vi "ControlPanelVI.vi"() -> ()   [LabVIEW 2024]
uses:
  <vilib>/Utility/error.llb/Trim Whitespace One-Sided.vi
  <vilib>/Instr/_visa.llb/VISA Configure Serial Port (Instr).vi
  <vilib>/regexp/Match Regular Expression.xnode
panel:
  out "CONTROL PANEL":enum32{" PAGE 1", "SERIAL PORT"}(tab)
  out "DOWN":u32(colorbox)
  out "-----":u32(colorbox)
  out "UP":u32(colorbox)
  out "Waveform Chart":u32(graph)
  out "on/off":u32(colorbox)=56405
  in  "SET ANGLE":i8(slide) min=-90 max=80 step=1 scale=-90.0..80.0
  out "Incline":i8(knob) scale=-90.0..80.0
  out "return count read":u32
  out "READ BUFFER":string
  in  "STOP":bool
  in  "milliseconds to wait":u32=1
  out "return count write":u32
  out "VISA resource name out read":refnum<visa-resource-name>="COM3"
  out "VISA resource name out write":refnum<visa-resource-name>="COM3"
  in  "send msg":bool
  in  "Safe Control":bool=TRUE
  out "input command":i8
  out "PWM (ms)":string
  out "DTC%":u8
  out "error out write":errorcluster
  out "error out read":errorcluster
  in  "VISA resource name":refnum<visa-resource-name>="COM3"
  in  "Enable Termination\nChar (T)":bool=TRUE
  in  "timeout (10sec)":u32=10000
  in  "baud rate (9600)":u32=9600
  in  "byte count":u32=100
  in  "parity (0:none)":enum16{"None", "Odd", "Even", "Mark", "Space"}(ring)
  in  "data bits (8)":u16=8 min=5 max=8 step=1
  in  "termination char\n(0xA = '\\n' = LF)":u8=10 format="%.0x"
  in  "flow control (0:none)":u16(ring)=3 items=["None", "XON/XOFF", "RTS/CTS", "XON/XOFF & RTS/CTS", "DTR/DSR", "XON/XOFF & DTR/DSR"]
  in  "stop bits (10: 1 bit)":u16(ring)=10 items=["1.0"=10, "1.5"=15, "2.0"=20]
  # "per = 20000"
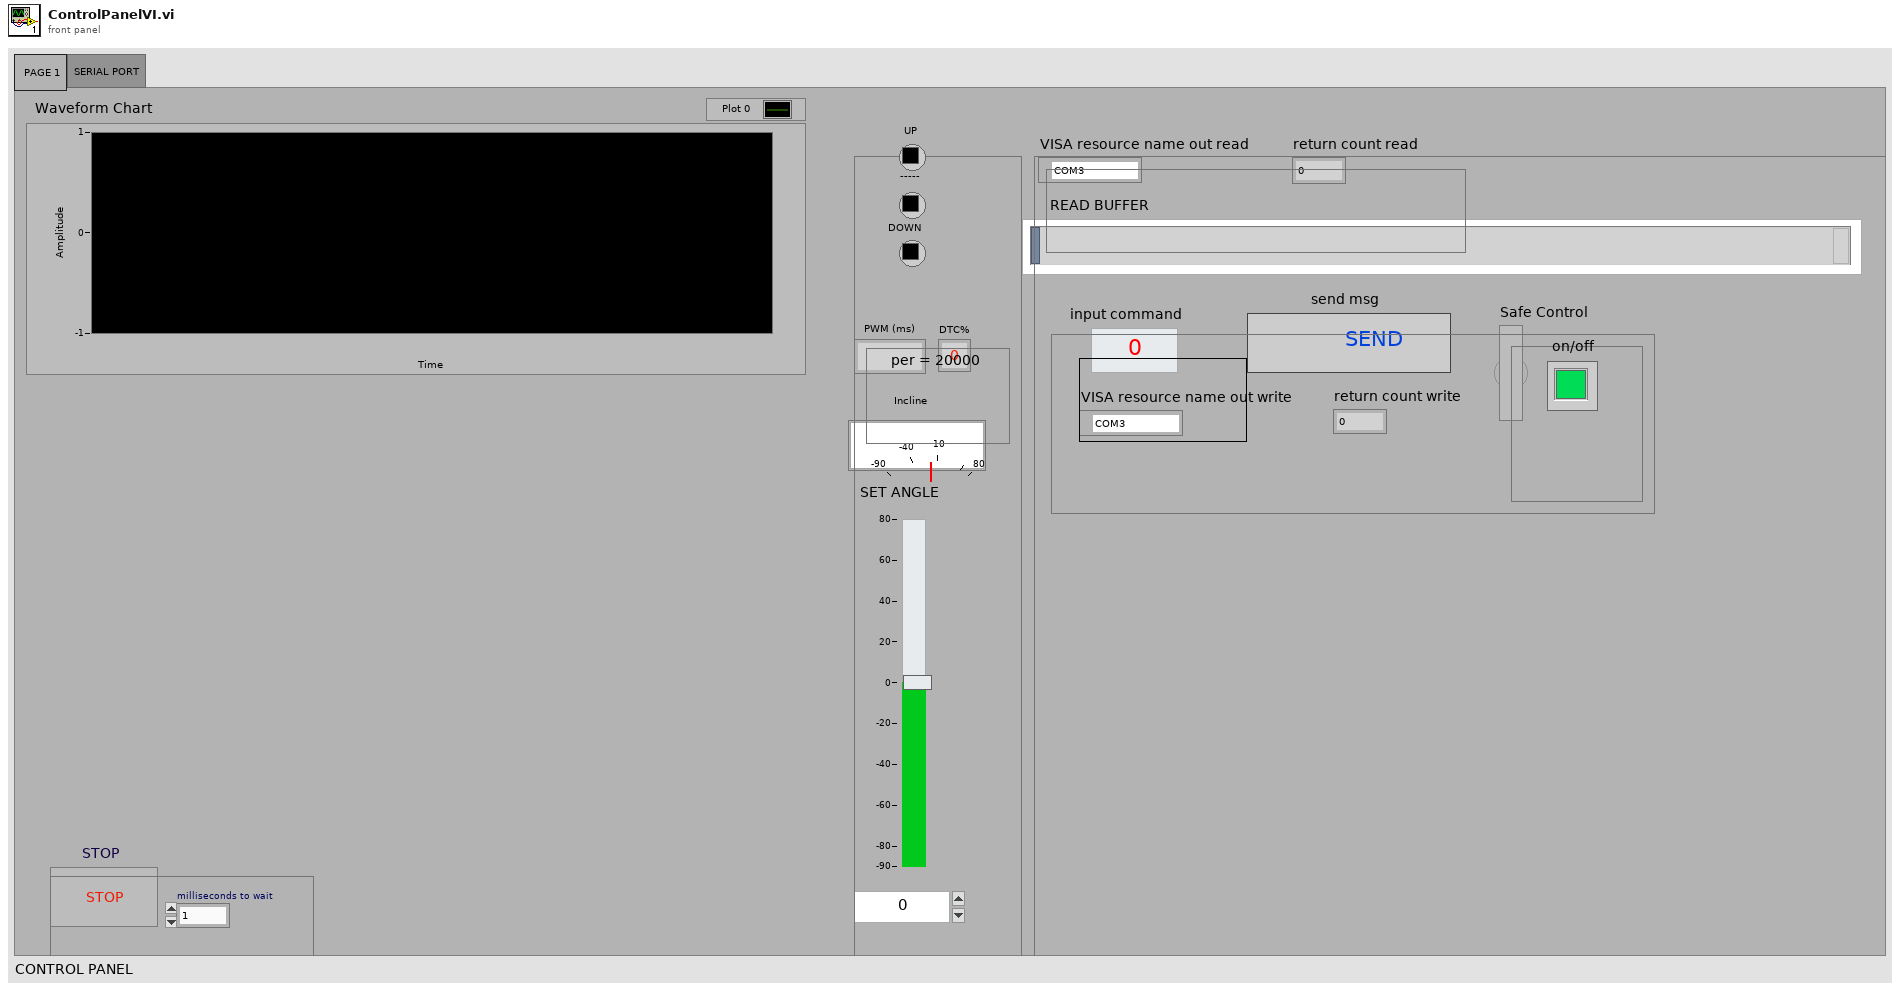
[diagram p1: front panel]
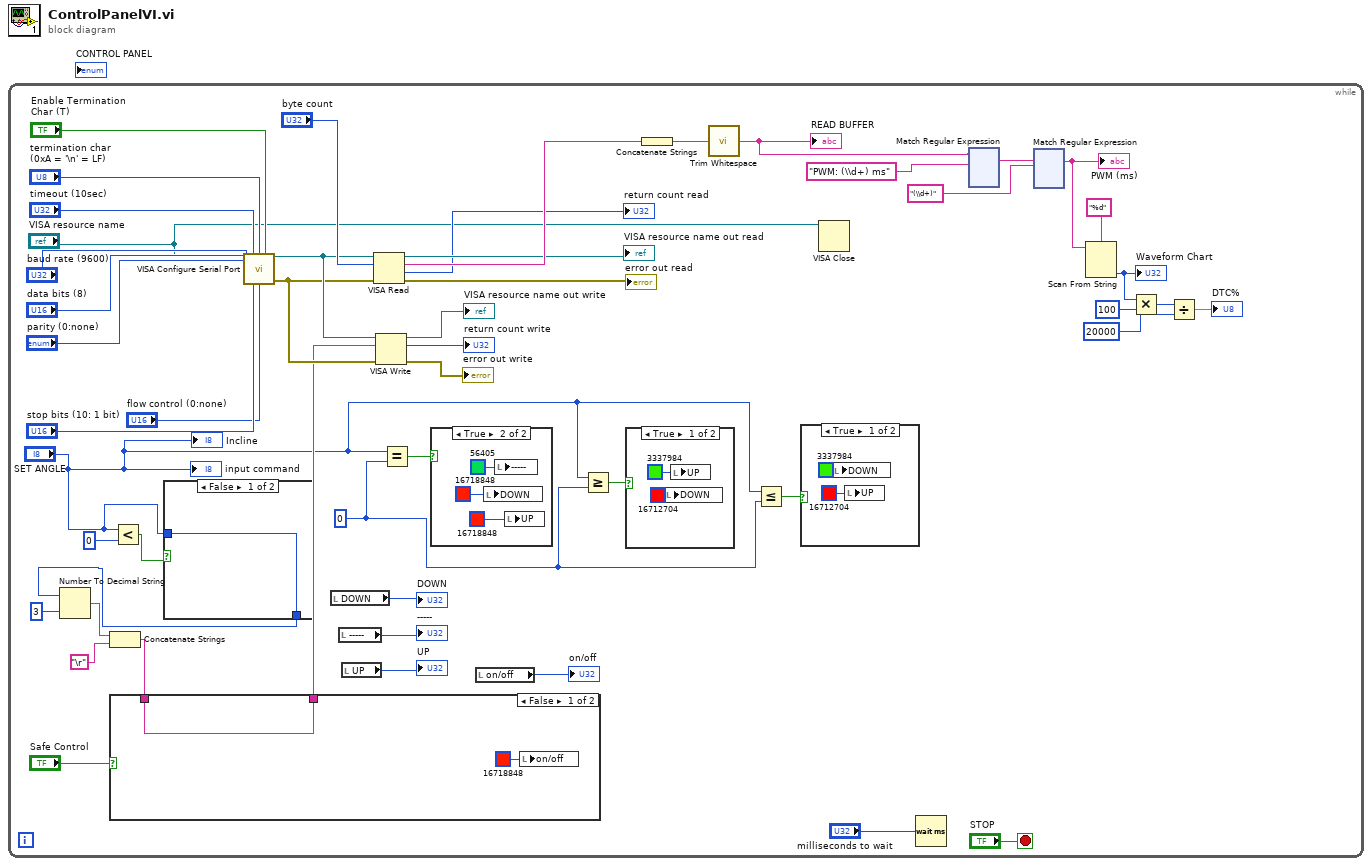
[diagram p0: block diagram]
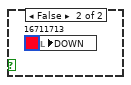
[diagram p2: hidden frame]
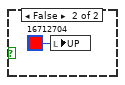
[diagram p3: hidden frame]
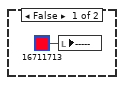
[diagram p4: hidden frame]
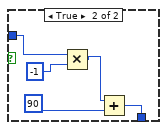
[diagram p5: hidden frame]
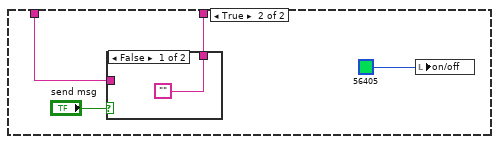
[diagram p6: hidden frame]
diagram:
  n1 = while {
    stop <- "STOP" stop-if-true
    w6 = i8 0 ("y")
    n2 = Less?(x="SET ANGLE", y=0) -> (x < y?=w22:bool)
    n3 = case shown="False" w22 {
      tunnel: "SET ANGLE" -> [w296 w298]
      tunnel: [w296 w300] -> w21
      frame False {
      }
      frame True {
        n4 = Multiply(x=w298, y=-1) -> (x*y=w299:i32)
        n5 = Add(x=w299, y=90) -> (x+y=w300:i32)
      }
    }
    n6 = Number To Decimal String(number=w21, width (-)=i16 3) -> (decimal integer string=w29:string)
    n7 = Concatenate Strings(w29, "\r" ("string")) -> (w26:string)
    n8 = case shown="False" "Safe Control" {
      tunnel: w26 -> [w303 w306]
      tunnel: [w303 w305] -> w25
      frame False {
        n9 = local write "on/off"(u32 16718848 ("on/off")) -> ()
      }
      frame True {
        n10 = case shown="False" "send msg" {
          tunnel: ["" w309] -> w305
          tunnel: w306 -> [_ w309]
          frame False {
          }
          frame True {
          }
        }
        n11 = local write "on/off"(u32 56405 ("on/off 2")) -> ()
      }
    }
    n12 = call-poly "VISA Configure Serial Port"("VISA resource name"="VISA resource name", "timeout (10sec)"="timeout (10sec)", "termination char\n(0xA = '\\n' = LF)"="termination char\n(0xA = '\\n' = LF)", "Enable Termination\nChar (T)"="Enable Termination\nChar (T)", "baud rate (9600)"="baud rate (9600)", "data bits (8)"="data bits (8)", "parity (0:none)"="parity (0:none)", "stop bits (10: 1 bit)"="stop bits (10: 1 bit)", "flow control (0:none)"="flow control (0:none)") -> ("VISA resource name out"=w42:refnum<visa-resource-name>, "error out"=w41:errorcluster)  [unwired: 5 in]
    n13 = local read "DOWN"() -> (→"DOWN":u32)
    n14 = local read "-----"() -> (→"-----":u32)
    n15 = local read "UP"() -> (→"UP":u32)
    n16 = VISA Read(VISA resource name=w42, byte count="byte count", error in (no error)=w41) -> (VISA resource name out=→"VISA resource name out read":refnum<visa-resource-name>, read buffer=w40:string, return count=→"return count read":u32, error out=→"error out read":errorcluster)
    n17 = VISA Write(VISA resource name=w42, write buffer=w25, error in (no error)=w41) -> (VISA resource name out=→"VISA resource name out write":refnum<visa-resource-name>, return count=→"return count write":u32, error out=→"error out write":errorcluster)
    n18 = Equal?(x="SET ANGLE", y=w6) -> (x = y?=w10:bool)
    n19 = case shown="True" w10 {
      frame False {
        n20 = local write "-----"(u32 16711713 ("-----")) -> ()
      }
      frame True {
        n21 = local write "DOWN"(u32 16718848 ("UP")) -> ()
        n22 = local write "-----"(u32 56405 ("-----")) -> ()
        n23 = local write "UP"(u32 16718848 ("DOWN")) -> ()
      }
    }
    n24 = local read "on/off"() -> (→"on/off":u32)
    n25 = Greater Or Equal?(x="SET ANGLE", y=w6) -> (x >= y?=w9:bool)
    n26 = case shown="True" w9 {
      frame True {
        n27 = local write "DOWN"(u32 16712704 ("UP")) -> ()
        n28 = local write "UP"(u32 3337984 ("UP")) -> ()
      }
      frame False {
        n29 = local write "UP"(u32 16712704 ("UP")) -> ()
      }
    }
    n30 = Concatenate Strings(w40) -> (w32:string)
    n31 = call <vilib>:"Trim Whitespace.vi"("string"=w32) -> ("trimmed string"=w19:string)  [unwired: 1 in]
    "READ BUFFER" <- w19
    n32 = Less Or Equal?(x="SET ANGLE", y=w6) -> (x <= y?=w8:bool)
    n33 = case shown="True" w8 {
      frame True {
        n34 = local write "DOWN"(u32 3337984 ("UP")) -> ()
        n35 = local write "UP"(u32 16712704 ("UP")) -> ()
      }
      frame False {
        n36 = local write "DOWN"(u32 16711713 ("UP")) -> ()
      }
    }
    n37 = VISA Close(VISA resource name="VISA resource name") -> ()  [unwired: 1 in, 1 out]
    n38 = Wait (ms)(milliseconds to wait="milliseconds to wait") -> ()  [unwired: 1 out]
    n39 = xnode "Match Regular Expression"("input string"=w19, "regular expression"="PWM: (\\d+) ms") -> ("whole match"=w16:string)  [unwired: 4 in, 4 out]
    n40 = xnode ("Match Regular Expression")("input string"=w16, "regular expression"="(\\d+)") -> ("whole match"=w14:string)  [unwired: 4 in, 4 out]
    "PWM (ms)" <- w14
    n41 = Scan From String "Scan From String"(format string="%d", input string=w14) -> (output 1=w5:u32)  [unwired: 3 in, 3 out]
    "Waveform Chart" <- w5
    n42 = Multiply(x=w5, y=u32 100) -> (x*y=w3:u32)
    n43 = Divide(x=w3, y=u32 20000) -> (x/y=→"DTC%":dbl)
    "Incline" <- "SET ANGLE"
    "input command" <- "SET ANGLE"
  }
